vi "kameravariabler.vi"() -> ()   [LabVIEW 2019]
panel:
  out "Pos right leg":dbl
  out "Pos left leg":dbl
  out "Pos Body":dbl
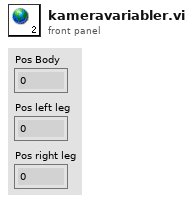
[diagram p1: front panel]
diagram:
